vi "插入数据.vi"(6 "error in (no error)":errorcluster, 8 "单条数据":T1, 11 "数据库连接引用 i":T2) -> (0 "error out":errorcluster, 3 "数据库连接引用 o":T2)   [LabVIEW 2017]
uses:
  <vilib>/addons/database/Connection.llb/Conn ObjectReference.ctl
  <vilib>/addons/database/NI_Database_API.lvlib
panel:
  out "Result":string caption="结果"
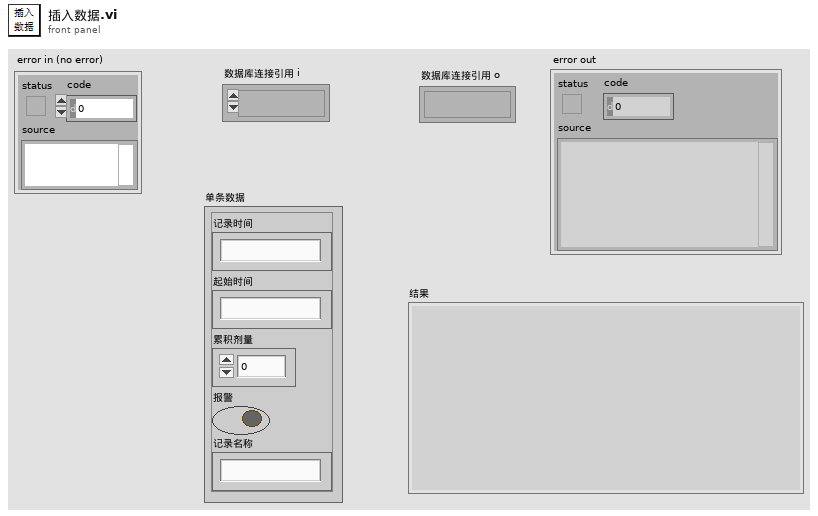
[diagram p1: front panel]
types:
  T1 = cluster{"记录时间":string, "起始时间":string, "累积剂量":dbl, "报警":bool, "记录名称":string}
  T2 = typedef "NI_Database_API.lvlib/Conn ObjectReference.ctl" = refnum<k1>
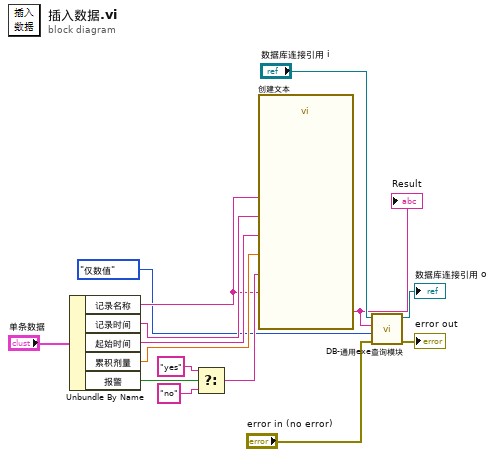
[diagram p0: block diagram]
diagram:
  n1 = Unbundle By Name("单条数据") -> ("记录名称"=w7:string, "记录时间"=w14:string, "起始时间"=w13:string, "累积剂量"=w12:dbl, "报警"=w9:bool)
  n2 = Select(t="yes", s=w9, f="no") -> (s? t:f=w8:string)
  n3 = call "创建文本"("累积剂量"=w12, "记录名称"=w7, "表名"=w7, "记录时间"=w14, "起始时间"=w13, "报警"=w8) -> ("Result"=w1:string)  [unwired: 8 in, 1 out]
  "Result" <- w1
  n4 = call "DB-通用exe查询模块.vi"("error in (no error)"="error in (no error)", "解析模式"=enum16{"仅数值", "仅字符串", "数值与字符串"}."仅数值", "SQL query"=w1, "数据库连接引用"="数据库连接引用 i") -> ("error out"=→"error out":errorcluster, "数据库连接引用out"=→"数据库连接引用 o":T2)  [unwired: 3 in, 3 out]
